vi "Convert Temperatures.vi"() -> ()   [LabVIEW 2012]
panel:
  out "Temperatures (Kelvin)":dbl[](array[numeric])
  in  "Temperatures (Celsius)":dbl[](array[numeric])=[-120.0, -200.0, -75.0, -45.0, -274.0]
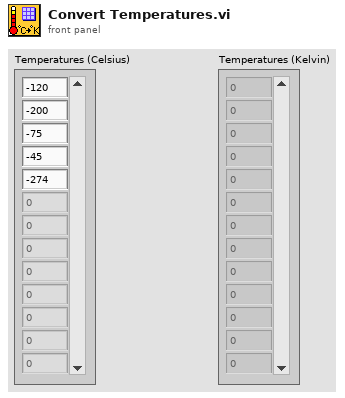
[diagram p1: front panel]
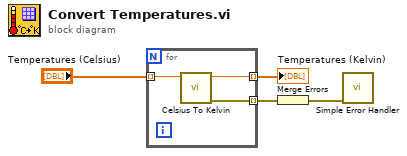
[diagram p0: block diagram]
diagram:
  n1 = for {
    tunnel: "Temperatures (Celsius)" -> [w7] mode=indexing
    tunnel: [w6] -> w3 mode=indexing
    tunnel: [w5] -> w2 mode=indexing
    n2 = call "Celsius To Kelvin.vi"("Celsius Value"=w7) -> ("error out"=w5:errorcluster, "Kelvin Value"=w6:dbl)  [unwired: 9 in]
  }
  "Temperatures (Kelvin)" <- w3
  n3 = Merge Errors(w2) -> (w1:errorcluster)
  n4 = call <vilib>:"Simple Error Handler.vi"("error in (no error)"=w1) -> ()  [unwired: 4 in, 5 out]
